vi "runTestScenario.vi"(8 "error in (no error)":errorcluster, 11 "EXC1Test in":refnum<class "EXC1Test.lvclass">) -> (0 "error out":errorcluster, 2 "TestExecution":T1, 3 "EXC1Test out":refnum<class "EXC1Test.lvclass">)   [LabVIEW 2015, in "EXC1Test.lvclass"]
uses:
  EXC1Test.lvclass
  Typedefs/TestExecution.ctl
  Typedefs/WriteDataFileInput.ctl
  Typedefs/TestScenarioTypes.ctl
  Typedefs/WriteLogMessageInput.ctl
  Typedefs/PassFailTest.ctl
  EXC1Test.lvclass/EXC1Test.ctl
  Model/TestLog/ITestLog/ITestLog.lvclass
  Typedefs/ILCBTTypedefs.lvlib
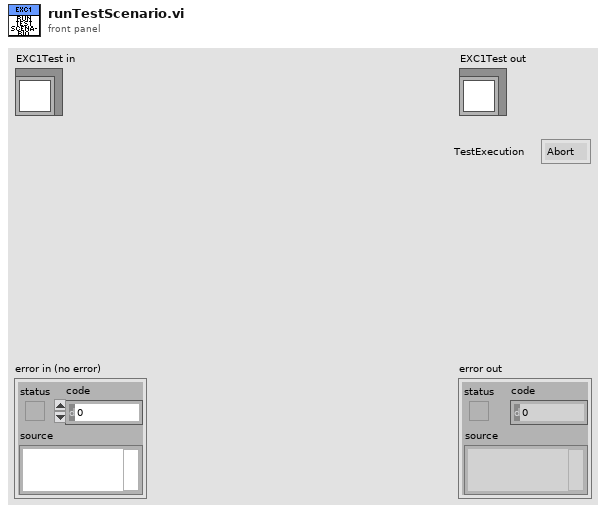
[diagram p1: front panel]
types:
  T1 = typedef "ILCBTTypedefs.lvlib/TestExecution.ctl" = enum16{"Abort", "Continue"}
  T2 = typedef "ILCBTTypedefs.lvlib/WriteLogMessageInput.ctl" = cluster{"Test Scenario":T3, "Description":string, "Actual Value":string, "Data File":string, "Result":T4}
  T3 = typedef "ILCBTTypedefs.lvlib/TestScenarioTypes.ctl" = enum16{"+3.3VA Supply Test", "+3.3VD Supply Test", "+5VA Supply Test", "+5VD Supply Test", "Unique ID Test", "TEDS Status Test", "LIMSW1_TTL Low Test", "LIMSW1_TTL High Test", "LIMSW2_TTL Low Test", "LIMSW2_TTL High Test", "Tachometer Test", "SSR_TTL Low Test", "SSR_TTL High Test", "SM_CW Low Test", "SM_CW High Test", "SM_CCW Low Test", "SM_CCW High Test", "SM_GPI Low Test", "SM_GPI High Test", "CW Motion Without Limit Test", "CW Motion With Limit Test", "CW Motion With Limit Interruption Test", "CW Motion on CCW Limit Test", "CCW Motion Without Limit Test", "CCW Motion With Limit Test", "CCW Motion With Limit Interruption Test", "CCW Motion on CW Limit Test", "RS232-TXD Low Test", "RS232-TXD High Test", "RS232-RTS Low Test", "RS232-RTS High Test", "RS232-RXD Low Test", "RS232-RXD High Test", "RS232-CTS Low Test", "RS232-CTS High Test", "Out_SS Low Test", "Out_SS High Test", "Out_SDI Low Test", "Out_SDI High Test", "Out_SCLK Low Test", "Out_SCLK High Test", "Reset Low Test", "Reset High Test", "1 Channel ADC Test", "3 Channel ADC Test", "5 Channel ADC Test", "Vref Test", "ROT Test", "DAC1 Test", "DAC2 Test", "DAC3 Test", "DAC4 Test", "BIAS Test", "EXC1 Test", "EXC2 Test", "EXC3 Test", "EXC4 Test"}
  T4 = typedef "ILCBTTypedefs.lvlib/PassFailTest.ctl" = enum16{"Fail", "Pass", "NA"}
  T5 = typedef "ILCBTTypedefs.lvlib/WriteDataFileInput.ctl" = cluster{"Test Scenario":T3, "File Name":string, "Output":dbl[]}
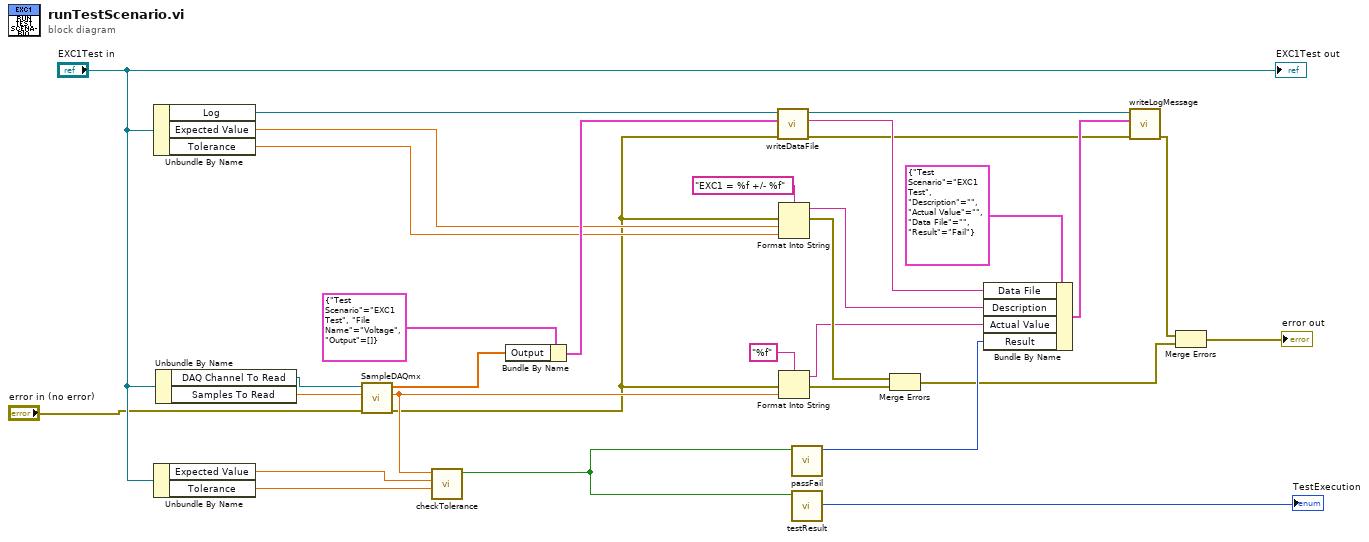
[diagram p0: block diagram]
diagram:
  n1 = Unbundle By Name("EXC1Test in") -> ("Log"=w31:refnum<class "ITestLog.lvclass">, "Expected Value"=w15:dbl[unit], "Tolerance"=w14:dbl[unit])
  n2 = Unbundle By Name("EXC1Test in") -> ("Expected Value"=w19:dbl[unit], "Tolerance"=w18:dbl[unit])
  n3 = Unbundle By Name("EXC1Test in") -> ("DAQ Channel To Read"=w23:refnum<k21>, "Samples To Read"=w22:dbl)
  n4 = call "SampleDAQmx.vi"("error in (no error)"="error in (no error)", "Samples To Read"=w22, "DAQ Channel To Read"=w23) -> ("error out"=w13:errorcluster, "Average"=w16:dbl, "Samples"=w30:dbl[])  [unwired: 6 in]
  n5 = call "checkTolerance.vi"("Tolerance"=w18, "Expected Value"=w19, "Average"=w16) -> ("Boolean"=w17:bool)  [unwired: 8 in]
  n6 = Bundle By Name(cluster=T5 {"Test Scenario"=enum."EXC1 Test", "File Name"="Voltage", "Output"=[]} ("WriteDataFileInput"), "Output"=w30) -> (w20:T5)
  n7 = call-dynamic "writeDataFile.vi"("error in (no error)"=w13, "WriteDataFileInput"=w20, "ITestLog in"=w31) -> ("error out"=w10:errorcluster, "Relative Path"=w12:string, "ITestLog out"=w25:refnum<class "ITestLog.lvclass">)  [unwired: 6 in]
  n8 = Format Into String(format string="EXC1 = %f +/- %f", error in=w13, w15, w14) -> (resulting string=w11:string, error out=w9:errorcluster)  [unwired: 1 in]
  n9 = Format Into String(format string="%f", error in=w13, w16) -> (resulting string=w5:string, error out=w8:errorcluster)  [unwired: 1 in]
  n10 = call "passFail.vi"("Boolean"=w17) -> ("Result"=w26:T4)  [unwired: 10 in]
  n11 = call "testResult.vi"("Boolean"=w17) -> ("TestExecution"=→"TestExecution":T1)  [unwired: 10 in]
  n12 = Merge Errors(w9, w8) -> (w6:errorcluster)
  n13 = Bundle By Name(cluster=T2 {"Test Scenario"=enum."EXC1 Test", "Description"="", "Actual Value"="", "Data File"="", "Result"=enum."Fail"} ("WriteLogMessageInput"), "Data File"=w12, "Description"=w11, "Actual Value"=w5, "Result"=w26) -> (w24:T2)
  n14 = call-dynamic "writeLogMessage.vi"("error in (no error)"=w10, "WriteLogMessageInput"=w24, "ITestLog in"=w25) -> ("error out"=w7:errorcluster)  [unwired: 7 in, 1 out]
  n15 = Merge Errors(w7, w6) -> (→"error out":errorcluster)
  "EXC1Test out" <- "EXC1Test in"
